vi "fromDevVarDoubleStringArray.vi"(1 "argin":cluster{"dvalue":dbl[], "svalue":string[]}) -> (0 "ArgIO":cluster{"num data":u8[], "str data":string[]})   [LabVIEW 2014, in "tango.lvlib"]
uses:
  tango.lvlib
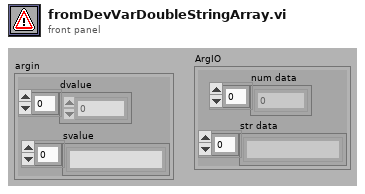
[diagram p1: front panel]
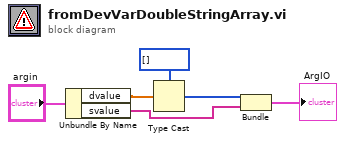
[diagram p0: block diagram]
diagram:
  n1 = Unbundle By Name("argin") -> ("dvalue"=w2:dbl[], "svalue"=w1:string[])
  n2 = Type Cast(type=u8[] [], x=w2) -> (*(type *) &x=w4:u8[])
  n3 = Bundle(w4, "svalue"=w1) -> (→"ArgIO":cluster{u8[], "svalue":string[]})  [unwired: 1 in]
